vi "Pin Position RowNames Read.vi"(4 "error in (no error)":errorcluster, 6 "Container State":T3, 7 "Display State In":T1) -> (0 "error out":errorcluster, 2 "Value":string[](array[string]), 3 "Display State Out":T1)   [LabVIEW 2013, in "Pin Position.xctl"]
uses:
  Pin Position.xctl
  <vilib>/_xctls/Container State.ctl
  Pin Position State.ctl
  lib/Data Access Objects/Application/Number Of LBCBs.ctl
  <vilib>/_xctls/XControlSupport.lvlib
panel:
  # "Replace the Value Indicator below with an Indicator of desired type.\nDo not remove this Indicator or the others from the connector pane. \nDo not change the connector pane pattern.\nThe Value Indicator should always be the second terminal from top on the output side in the connector pane."
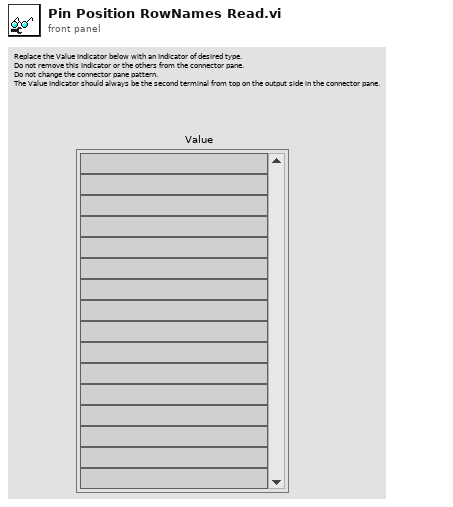
[diagram p1: front panel]
types:
  T1 = typedef "Pin Position.xctl/Pin Position State.ctl" = cluster{"Number  of LBCBs":T2, "RowNames":string[]}
  T2 = typedef "Number Of LBCBs.ctl" = enum16{"1", "2"}
  T3 = typedef "XControlSupport.lvlib/Container State.ctl" = cluster{"Indicator?":bool, "Run Mode?":bool, " Refnum":refnum<vi>}
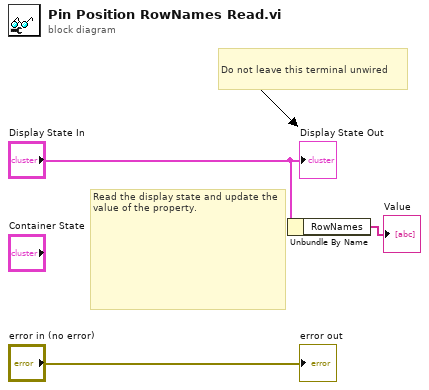
[diagram p0: block diagram]
diagram:
  # "Do not leave this terminal unwired"
  # "Read the display state and update the value of the property."
  n1 = Unbundle By Name("Display State In") -> ("RowNames"=→"Value":string[])
  "error out" <- "error in (no error)"
  "Display State Out" <- "Display State In"
